vi "Read Data Titles.vi"(8 "error in (no error)":errorcluster, 11 "HP53181 in":refnum<class "HP53181.lvclass">) -> (0 "error out":errorcluster, 2 "Data titles":string[](array[string])=["HP53181_Frequency (Hz)"], 3 "HP53181 out":refnum<class "HP53181.lvclass">)   [LabVIEW 2015, in "HP53181.lvclass"]
uses:
  HP53181.lvclass
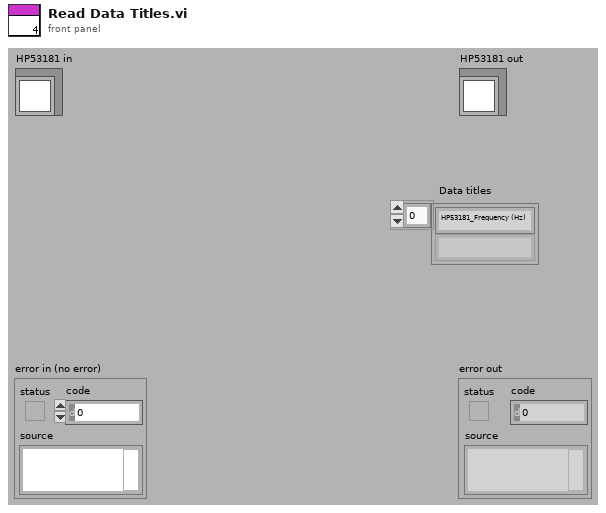
[diagram p1: front panel]
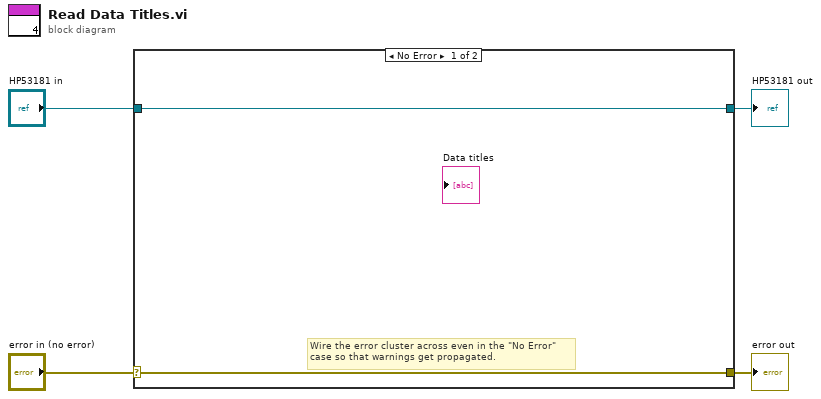
[diagram p0: block diagram]
diagram:
  n1 = case shown="No Error" "error in (no error)" {
    selector: "error in (no error)" -> [w5 w8]
    tunnel: [w5 w8] -> w3
    tunnel: [w6 w7] -> w1
    tunnel: "HP53181 in" -> [w6 w7]
    frame No Error {
      # "Wire the error cluster across even in the \"No Error\"\ncase so that warnings get propagated."
    }
    frame Error {
    }
  }
  "error out" <- w3
  "HP53181 out" <- w1
